vi "CD Init_Prepare Inline Data_Fill Broadcast Frame Descriptors from BC configuration.vi"(8 "error in (no error)":errorcluster, 11 "RT Channel In":T9 {"RTs"."Mode Codes"."Words Item Refs" format="%.0x"; "RTs"."Mode Codes"."Words Block Data Refs"."Data Reference" format="%.0x"; "RTs"."Mode Codes"."Timestamp Channel Data Reference" format="%.0x"; "RTs"."subAddresses"."Words Item Refs" format="%.0x"; "RTs"."subAddresses"."Words Block Data Refs"."Data Reference" format="%.0x"; "RTs"."subAddresses"."Timestamp Channel Data Reference" format="%.0x"; "RTs"."Status Channel Data Reference" format="%.0x"; "RTs"."Command Channels Refs" format="%.0x"; "BC"."Acyclic Frames Trigger Channels Refs" format="%.0x"; "BC"."Command Channels Refs" format="%.0x"; "BC"."messages"."Timestamp Channel Data Reference" format="%.0x"; "BC"."messages"."Status Channel Data Refs" format="%.0x"; "BC"."messages"."Words Item Refs" format="%.0x"; "BC"."messages"."Words Block Data Refs"."Data Reference" format="%.0x"}) -> (0 "error out":errorcluster, 1 "Broadcast Frame Descriptors Out":T15[](array[typedef]) {"RTs"."Status Channel Ref" format="%.0x"; "RTs"."Words Block Data Refs"."Data Reference" format="%.0x"; "RTs"."Timestamp Channel Data Reference" format="%.0x"; "BC"."Status Channel Refs" format="%.0x"; "BC"."Words Block Data Refs"."Data Reference" format="%.0x"; "BC"."Timestamp Channel Data Reference" format="%.0x"}, 2 "RTs Out":T1[](array[typedef]) {"Mode Codes"."Words Item Refs" format="%.0x"; "Mode Codes"."Words Block Data Refs"."Data Reference" format="%.0x"; "Mode Codes"."Timestamp Channel Data Reference" format="%.0x"; "subAddresses"."Words Item Refs" format="%.0x"; "subAddresses"."Words Block Data Refs"."Data Reference" format="%.0x"; "subAddresses"."Timestamp Channel Data Reference" format="%.0x"; "Status Channel Data Reference" format="%.0x"; "Command Channels Refs" format="%.0x"}, 3 "RT Channel Out":T9 {"RTs"."Mode Codes"."Words Item Refs" format="%.0x"; "RTs"."Mode Codes"."Words Block Data Refs"."Data Reference" format="%.0x"; "RTs"."Mode Codes"."Timestamp Channel Data Reference" format="%.0x"; "RTs"."subAddresses"."Words Item Refs" format="%.0x"; "RTs"."subAddresses"."Words Block Data Refs"."Data Reference" format="%.0x"; "RTs"."subAddresses"."Timestamp Channel Data Reference" format="%.0x"; "RTs"."Status Channel Data Reference" format="%.0x"; "RTs"."Command Channels Refs" format="%.0x"; "BC"."Acyclic Frames Trigger Channels Refs" format="%.0x"; "BC"."Command Channels Refs" format="%.0x"; "BC"."messages"."Timestamp Channel Data Reference" format="%.0x"; "BC"."messages"."Status Channel Data Refs" format="%.0x"; "BC"."messages"."Words Item Refs" format="%.0x"; "BC"."messages"."Words Block Data Refs"."Data Reference" format="%.0x"})   [LabVIEW 2017, in "Ballard MIL-1553 Engine.lvlib"]
uses:
  Ballard MIL-1553 Engine.lvlib
  Shared/Controls and Global/RT Channel.ctl
  Shared/Controls and Global/RT BC.ctl
  <vilib>/NI Veristand/Custom Device API/Custom Device Item Ref.ctl
  Shared/Controls and Global/RT Message.ctl
  Shared/Controls and Global/RT messageType.ctl
  Shared/Controls and Global/RT CWD1.ctl
  Shared/Controls and Global/RT CWD2.ctl
  <vilib>/NI Veristand/Custom Device API/Data Reference.ctl
  <vilib>/NI Veristand/Custom Device API/Block Data Reference.ctl
  Shared/Controls and Global/RT Remote Terminal.ctl
  Shared/Controls and Global/RT Remote Terminal_rtMode.ctl
  Shared/Controls and Global/RT Remote Terminal_RT subAddress.ctl
  Shared/Controls and Global/RT Remote Terminal_RT direction.ctl
  Shared/Controls and Global/RT Remote Terminal_RT Mode Code.ctl
  Controls/RT Inline Broadcast Frame Descriptor.ctl
  Controls/RT Inline Frame Descriptor_BC.ctl
  Controls/RT Inline Frame Descriptor_RT.ctl
  Shared/Ballard 1553 Shared.lvlib
  <vilib>/NI VeriStand/Custom Device API/Custom Device API.lvlib
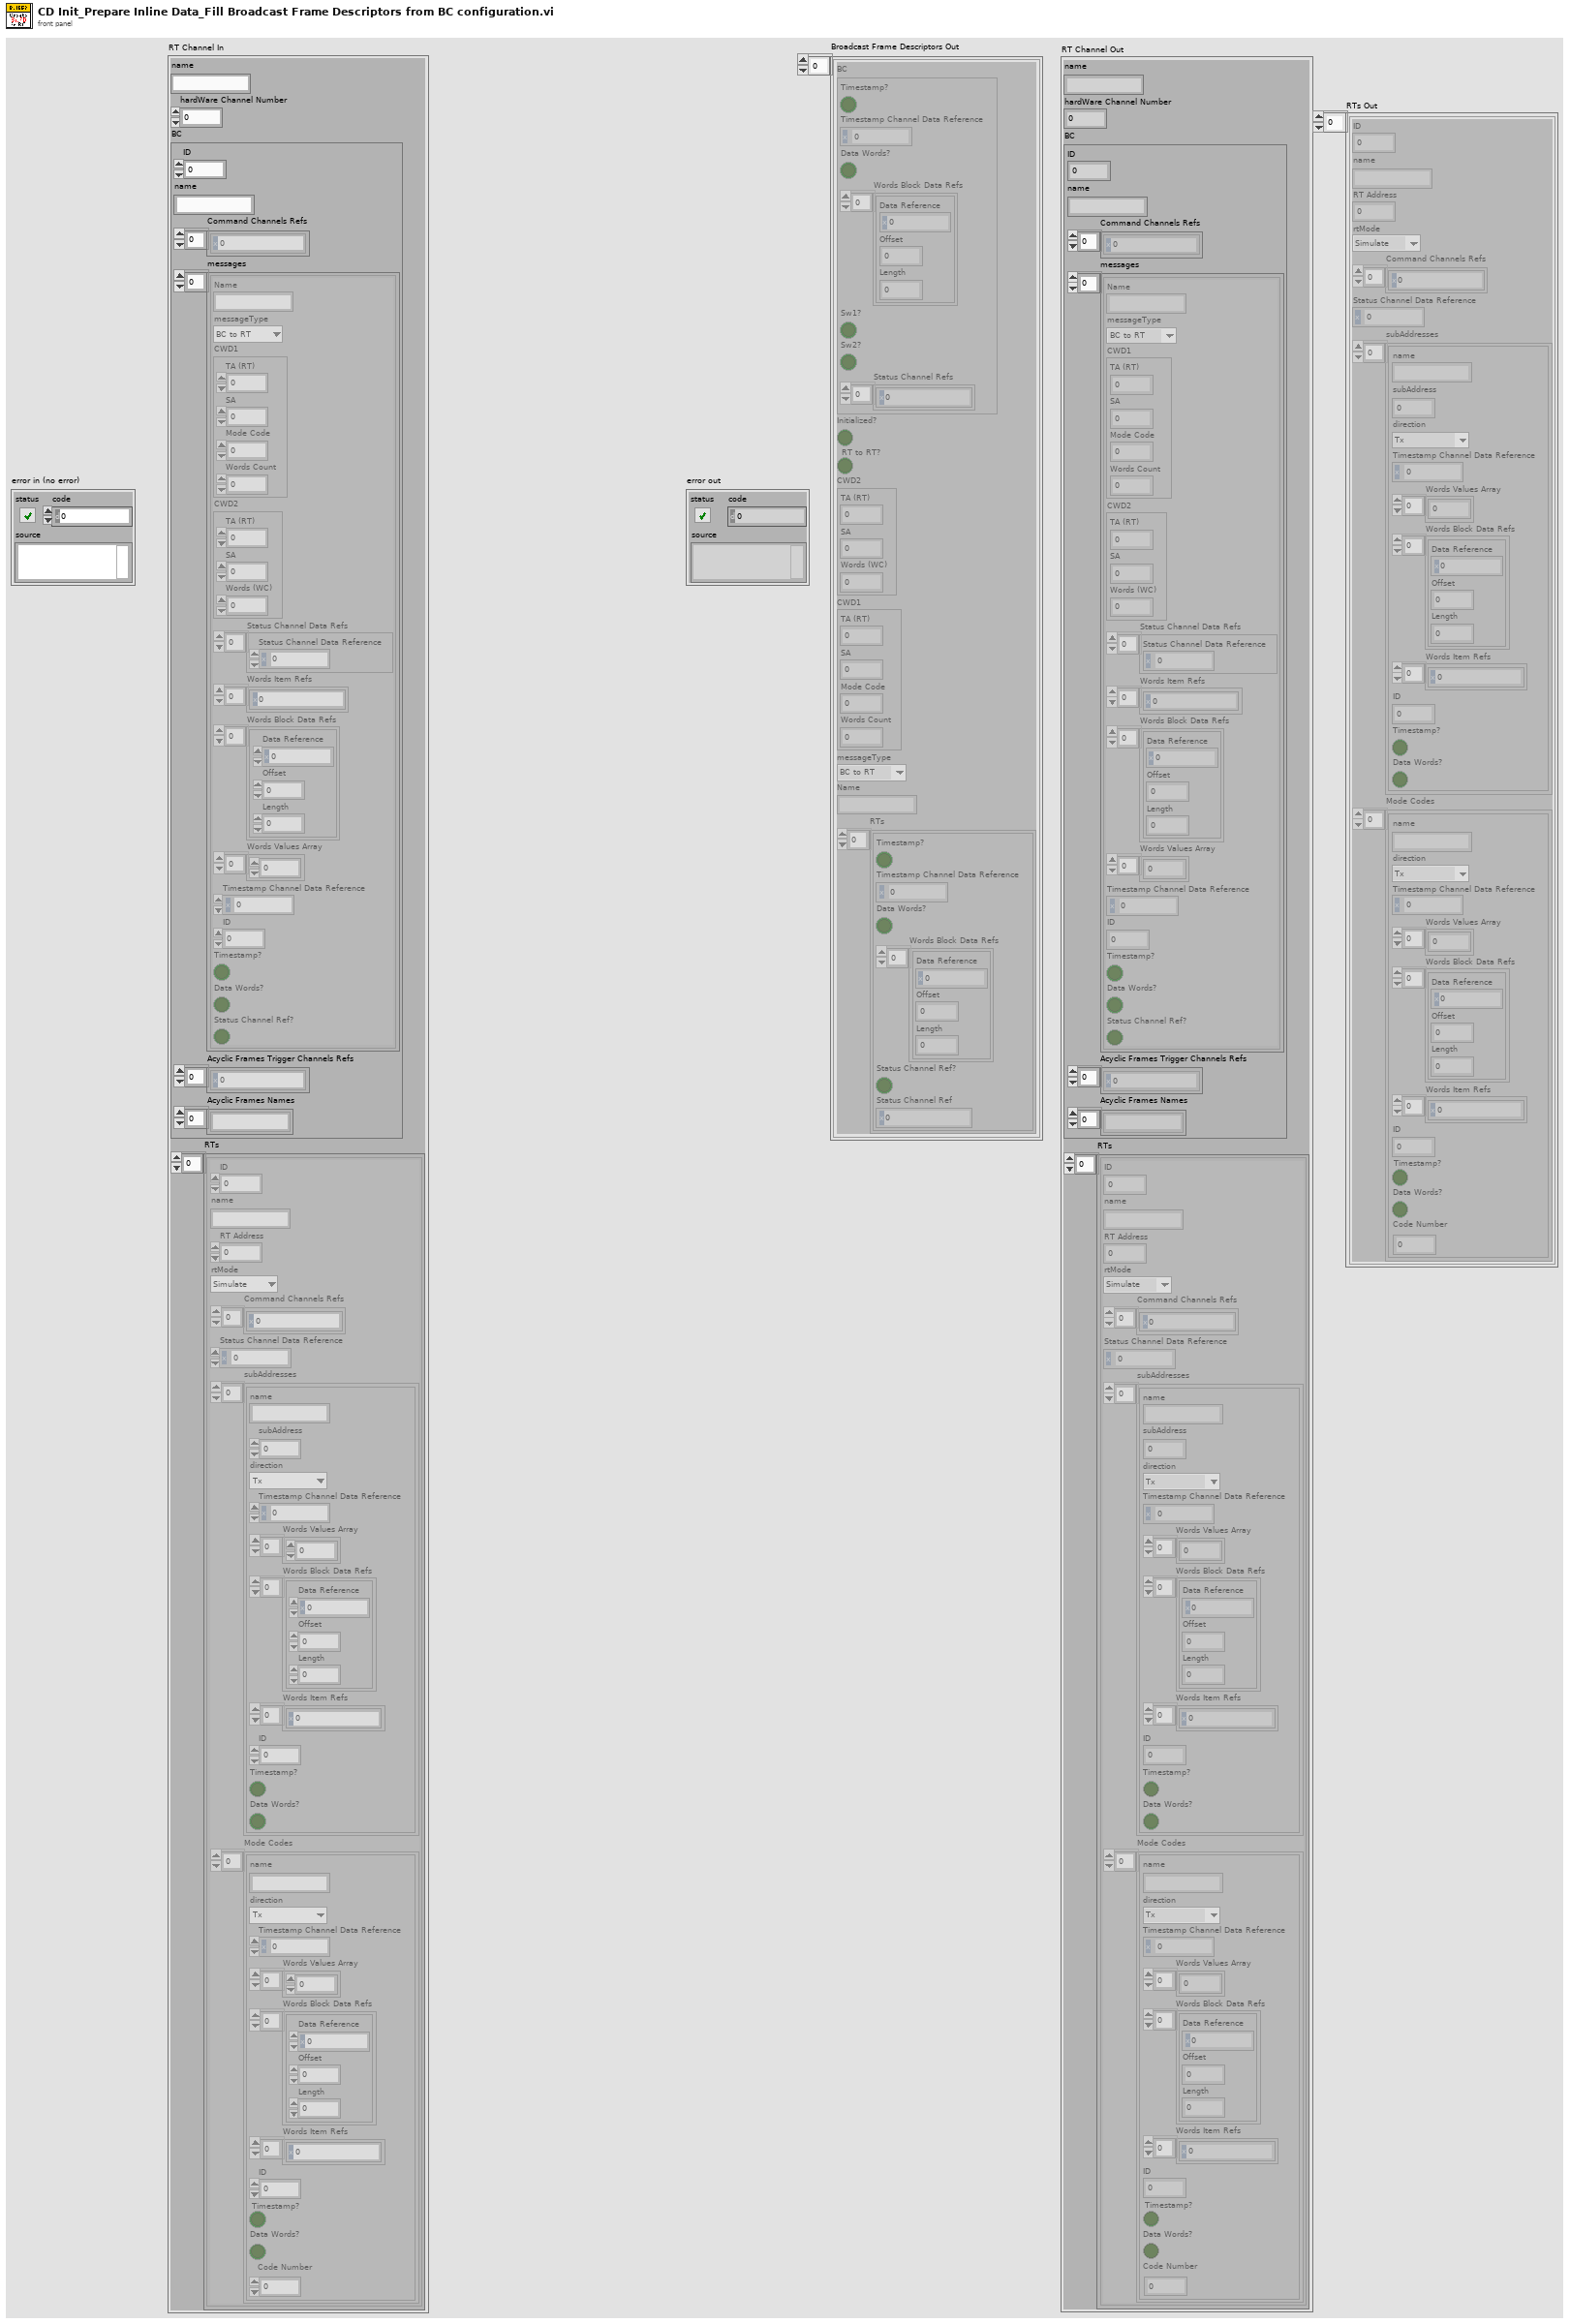
[diagram p1: front panel]
types:
  T1 = typedef "Ballard 1553 Shared.lvlib/RT Remote Terminal.ctl" = cluster{"ID":i32, "name":string, "RT Address":i32, "rtMode":T2, "Command Channels Refs":T3[], "Status Channel Data Reference":T4, "subAddresses":T5[], "Mode Codes":T8[]}
  T2 = typedef "Ballard 1553 Shared.lvlib/RT Remote Terminal_rtMode.ctl" = enum16{"Simulate", "Monitor", "Disable"}
  T3 = typedef "Custom Device API.lvlib/Custom Device Item Ref.ctl" = u64
  T4 = typedef "Custom Device API.lvlib/Data Reference.ctl" = i32
  T5 = typedef "Ballard 1553 Shared.lvlib/RT Remote Terminal_RT subAddress.ctl" = cluster{"name":string, "subAddress":i8, "direction":T6, "Timestamp Channel Data Reference":T4, "Words Values Array":u16[], "Words Block Data Refs":T7[], "Words Item Refs":T3[], "ID":i32, "Timestamp?":bool, "Data Words?":bool}
  T6 = typedef "Ballard 1553 Shared.lvlib/RT Remote Terminal_RT direction.ctl" = enum16{"Tx", "Rx"}
  T7 = typedef "Custom Device API.lvlib/Block Data Reference.ctl" = cluster{"Data Reference":T4, "Offset":u64, "Length":u64}
  T8 = typedef "Ballard 1553 Shared.lvlib/RT Remote Terminal_RT Mode Code.ctl" = cluster{"name":string, "direction":T6, "Timestamp Channel Data Reference":T4, "Words Values Array":u16[], "Words Block Data Refs":T7[], "Words Item Refs":T3[], "ID":i32, "Timestamp?":bool, "Data Words?":bool, "Code Number":i32}
  T9 = typedef "Ballard 1553 Shared.lvlib/RT Channel.ctl" = cluster{"name":string, "hardWare Channel Number":u16, "BC":T10, "RTs":T1[]}
  T10 = typedef "Ballard 1553 Shared.lvlib/RT BC.ctl" = cluster{"ID":i32, "name":string, "Command Channels Refs":T3[], "messages":T11[], "Acyclic Frames Trigger Channels Refs":T3[], "Acyclic Frames Names":string[]}
  T11 = typedef "Ballard 1553 Shared.lvlib/RT Message.ctl" = cluster{"Name":string, "messageType":T12, "CWD1":T13, "CWD2":T14, "Status Channel Data Refs":T4[], "Words Item Refs":T3[], "Words Block Data Refs":T7[], "Words Values Array":u16[], "Timestamp Channel Data Reference":T4, "ID":i32, "Timestamp?":bool, "Data Words?":bool, "Status Channel Ref?":bool}
  T12 = typedef "Ballard 1553 Shared.lvlib/RT messageType.ctl" = enum16{"BC to RT", "RT to BC", "RT to RT", "MC (Rx)", "MC (Tx)"}
  T13 = typedef "Ballard 1553 Shared.lvlib/RT CWD1.ctl" = cluster{"TA (RT)":i8, "SA":i8, "Mode Code":i8, "Words Count":i8}
  T14 = typedef "Ballard 1553 Shared.lvlib/RT CWD2.ctl" = cluster{"TA (RT)":i8, "SA":i8, "Words (WC)":i8}
  T15 = typedef "Ballard MIL-1553 Engine.lvlib/RT Inline Broadcast Frame Descriptor.ctl" = cluster{"BC":T16, "Initialized?":bool, "RT to RT?":bool, "CWD2":T14, "CWD1":T13, "messageType":T12, "Name":string, "RTs":T17[]}
  T16 = typedef "Ballard MIL-1553 Engine.lvlib/RT Inline Frame Descriptor_BC.ctl" = cluster{"Timestamp?":bool, "Timestamp Channel Data Reference":T4, "Data Words?":bool, "Words Block Data Refs":T7[], "Sw1?":bool, "Sw2?":bool, "Status Channel Refs":T3[]}
  T17 = typedef "Ballard MIL-1553 Engine.lvlib/RT Inline Frame Descriptor_RT.ctl" = cluster{"Timestamp?":bool, "Timestamp Channel Data Reference":T4, "Data Words?":bool, "Words Block Data Refs":T7[], "Status Channel Ref?":bool, "Status Channel Ref":T3}
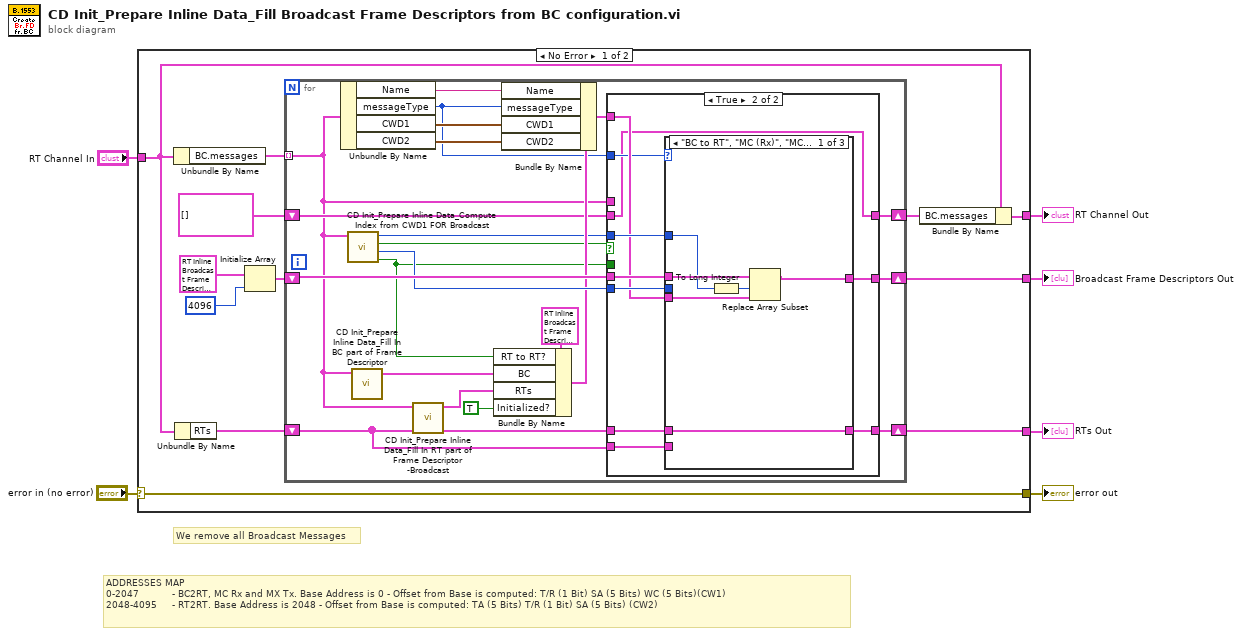
[diagram p0: block diagram]
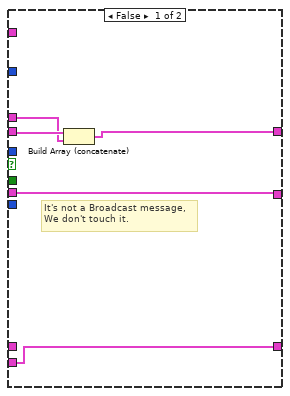
[diagram p2: hidden frame]
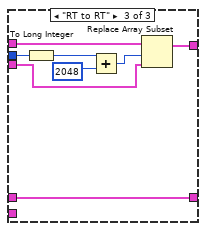
[diagram p4: hidden frame]
diagram:
  # "We remove all Broadcast Messages"
  # "ADDRESSES MAP \n0-2047           - BC2RT, MC Rx and MX Tx. Base Address is 0 - Offset from Base is computed: T/R (1 Bit) SA (5 Bits) WC (5 Bits)(CW1)\n2048-4095     - RT2RT. Base Address is 2048 - Offset from Base is computed: TA (5 Bits) T/R (1 Bit) SA (5 Bits) (CW2)"
  n1 = case shown="No Error" "error in (no error)" {
    selector: "error in (no error)" -> [w14 w73]
    tunnel: [w17 _] -> w2
    tunnel: "RT Channel In" -> [w12 w72]
    tunnel: [w14 w73] -> w4
    tunnel: [w10 w72] -> w3
    tunnel: [w7 _] -> w1
    frame No Error {
      n2 = Unbundle By Name(w12) -> ("BC.messages"=w9:T11[])
      n3 = Unbundle By Name(w12) -> ("RTs"=w13:T1[])
      n4 = Initialize Array(T15 {"BC"={"Timestamp?"=FALSE, "Timestamp Channel Data Reference"=0, "Data Words?"=FALSE, "Words Block Data Refs"=[], "Sw1?"=FALSE, "Sw2?"=FALSE, "Status Channel Refs"=[]}, "Initialized?"=FALSE, "RT to RT?"=FALSE, "CWD2"={"TA (RT)"=0, "SA"=0, "Words (WC)"=0}, "CWD1"={"TA (RT)"=0, "SA"=0, "Mode Code"=0, "Words Count"=0}, "messageType"=enum."BC to RT", "Name"="", "RTs"=[]} ("Frame Descriptor"), 4096 ("dimension size")) -> (w16:T15[])
      n5 = for {
        shift-right: [w39] -> w17
        shift-left: w16 -> [w40]
        shift-right: [w24] -> w11
        shift-left: T11[] [] -> [w26]
        tunnel: w9 -> [w25] mode=indexing
        shift-right: [w20] -> w7
        shift-left: w13 -> [w21]
        n6 = Unbundle By Name(w25) -> ("Name"=w34:string, "messageType"=w27:T12, "CWD1"=w33:T13, "CWD2"=w32:T14)
        n7 = call "CD Init_Prepare Inline Data_Compute Index from CWD1 FOR Broadcast.vi"("message"=w25) -> ("RT to RT?"=w29:bool, "Index 1"=w36:u32, "Broadcast?"=w28:bool, "Index 0"=w31:u16)  [unwired: 6 in, 1 out]
        n8 = call "CD Init_Prepare Inline Data_Fill In BC part of Frame Descriptor.vi"("message"=w25) -> ("BC Frame Descriptor"=w38:T16)  [unwired: 10 in]
        n9 = call "CD Init_Prepare Inline Data_Fill In RT part of Frame Descriptor -Broadcast.vi"("RTs In"=w21, "message"=w25) -> ("RTs Out"=w19:T1[], "RTs Frame Descriptors"=w22:T17[])  [unwired: 8 in]
        n10 = Bundle By Name(cluster=T15 {"BC"={"Timestamp?"=FALSE, "Timestamp Channel Data Reference"=0, "Data Words?"=FALSE, "Words Block Data Refs"=[], "Sw1?"=FALSE, "Sw2?"=FALSE, "Status Channel Refs"=[]}, "Initialized?"=FALSE, "RT to RT?"=FALSE, "CWD2"={"TA (RT)"=0, "SA"=0, "Words (WC)"=0}, "CWD1"={"TA (RT)"=0, "SA"=0, "Mode Code"=0, "Words Count"=0}, "messageType"=enum."BC to RT", "Name"="", "RTs"=[]} ("Frame Descriptor"), "RT to RT?"=w29, "BC"=w38, "RTs"=w22, "Initialized?"=TRUE) -> (w35:T15)
        n11 = Bundle By Name(cluster=w35, "Name"=w34, "messageType"=w27, "CWD1"=w33, "CWD2"=w32) -> (w30:T15)
        n12 = case shown="True" w28 {
          tunnel: w40 -> [w45 w55]
          tunnel: [w45 w54] -> w39
          tunnel: w36 -> [_ w53]
          tunnel: w31 -> [_ w52]
          tunnel: w30 -> [_ w51]
          tunnel: w29 -> [_ _]
          tunnel: w27 -> [_ w50]
          tunnel: w26 -> [w44 w49]
          tunnel: w25 -> [w43 _]
          tunnel: [w42 w49] -> w24
          tunnel: w21 -> [w41 w48]
          tunnel: [w41 w47] -> w20
          tunnel: w19 -> [_ w46]
          frame False {
            # "It's not a Broadcast message,\nWe don't touch it."
            n13 = Build Array (concatenate)(w44, w43) -> (w42:T11[])
          }
          frame True {
            n14 = case shown="\"BC to RT\", \"MC (Rx)\", \"MC (Tx)\", Default" w50 {
              tunnel: w55 -> [w61 w63 w71]
              tunnel: [w60 w63 w70] -> w54
              tunnel: w53 -> [_ _ w67]
              tunnel: w51 -> [w57 _ w65]
              tunnel: w52 -> [w58 _ _]
              tunnel: w48 -> [_ w62 _]
              tunnel: [w56 w62 w64] -> w47
              tunnel: w46 -> [w56 _ w64]
              frame "BC to RT", "MC (Rx)", "MC (Tx)", Default {
                n15 = To Long Integer(number=w58) -> (32bit integer=w59:i32)
                n16 = Replace Array Subset(array=w61, new element=w57, index=w59) -> (w60:T15[])
              }
              frame "RT to BC" {
                # "Impossible case."
              }
              frame "RT to RT" {
                n17 = To Long Integer(number=w67) -> (32bit integer=w69:i32)
                n18 = Add(x=w69, y=2048) -> (x+y=w68:i32)
                n19 = Replace Array Subset(array=w71, new element=w65, index=w68) -> (w70:T15[])
              }
            }
          }
        }
      }
      n20 = Bundle By Name(cluster=w12, "BC.messages"=w11) -> (w10:T9)
    }
    frame Error {
    }
  }
  "error out" <- w4
  "Broadcast Frame Descriptors Out" <- w2
  "RT Channel Out" <- w3
  "RTs Out" <- w1
